vi "Choose configuration mode.vi"(8 "error in (no error)":errorcluster, 10 "Choose configuration mode":u16=65535, 11 "PS Control Actor in":refnum<class "PS Control Actor.lvclass">) -> (0 "error out":errorcluster, 3 "PS Control Actor out":refnum<class "PS Control Actor.lvclass">)   [LabVIEW 2025, in "PS Control Actor.lvlib" / "PS Control Actor.lvclass"]
doc: "Author: Scott Hannahs <sth@magnet.fsu.edu>\n\nThis software is licensed for use under the “MIT License\"\nCopyright (c) 2025 Scott Hannahs, sth@sth@magnet.sthnet.net\n\nPermission is hereby granted, free of charge, to any person obtaining a copy of this software and associated documentation files (the \"Software\"), to deal in the Software without restriction, including without limitation the rights to use, copy, modify, merge, publish, distribute, sublicense, and/or sell copies of the Software, and to permit persons to whom the Software is furnished to do so, subject to the following conditions: The above copyright notice and this permission notice shall be included in all copies or substantial portions of the Software.\n\nTHE SOFTWARE IS PROVIDED \"AS IS\", WITHOUT WARRANTY OF ANY KIND, EXPRESS OR IMPLIED, INCLUDING BUT NOT LIMITED TO THE WARRANTIES OF MERCHANTABILITY, FITNESS FOR A PARTICULAR PURPOSE AND NONINFRINGEMENT. IN NO EVENT SHALL THE AUTHORS OR COPYRIGHT HOLDERS BE LIABLE FOR ANY CLAIM, DAMAGES OR OTHER LIABILITY, WHETHER IN AN ACTION OF CONTRACT, TORT OR OTHERWISE, ARISING FROM, OUT OF OR IN CONNECTION WITH THE SOFTWARE OR THE USE OR OTHER DEALINGS IN THE SOFTWARE."
uses:
  PS Control Actor.lvclass
  PS Control Actor.lvclass/PS Control Actor.ctl
  PS Driver/PS Driver.lvclass
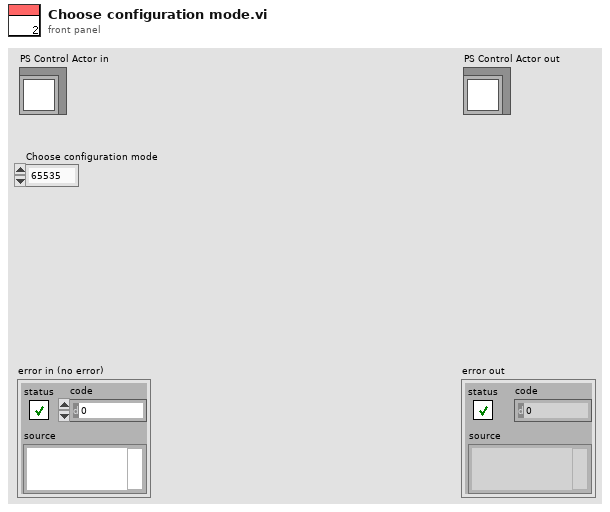
[diagram p1: front panel]
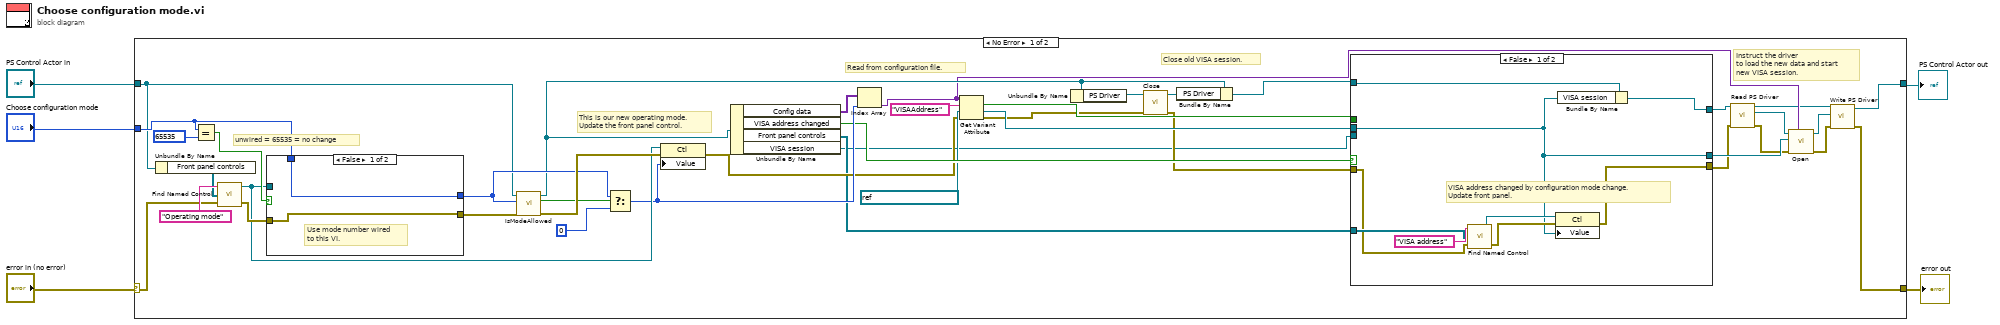
[diagram p0: block diagram]
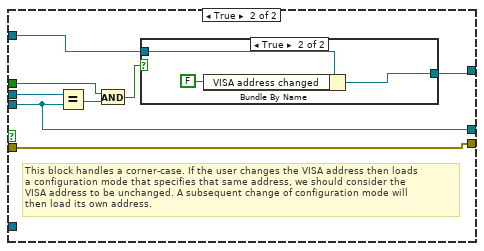
[diagram p2: hidden frame]
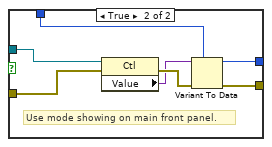
[diagram p4: hidden frame]
diagram:
  n1 = case shown="No Error" "error in (no error)" {
    selector: "error in (no error)" -> [w35 w78]
    tunnel: [w13 w78] -> w4
    tunnel: [w7 w77] -> w1
    tunnel: "PS Control Actor in" -> [w34 w77]
    tunnel: "Choose configuration mode" -> [w42 _]
    frame No Error {
      # "Close old VISA session."
      # "Read from configuration file."
      # "Instruct the driver \nto load the new data and start\nnew VISA session."
      # "This is our new operating mode.\nUpdate the front panel control."
      # "unwired = 65535 = no change"
      n2 = Unbundle By Name(w34) -> ("Front panel controls"=w33:refnum<vi>[])
      n3 = Equal?(x=w42, y=u16 65535) -> (x = y?=w45:bool)
      n4 = call "Find Named Control.vi"("error in"=w35, "All Controls"=w33, "Control Name"="Operating mode") -> ("error out"=w43:errorcluster, "Ctl Refnum"=w36:refnum<vi>)  [unwired: 1 out]
      n5 = case shown="False" w45 {
        tunnel: [w68 w74] -> w39
        tunnel: [w69 w73] -> w41
        tunnel: w43 -> [w69 w72]
        tunnel: w36 -> [_ w71]
        tunnel: w42 -> [w68 w70]
        frame False {
          # "Use mode number wired\nto this VI."
        }
        frame True {
          # "Use mode showing on main front panel."
          n6 = property class="Ctl"(reference=w71, error in=w72) -> (error out=w76:errorcluster, "Value"=w75:variant)  [unwired: 1 out]
          n7 = Variant To Data(error in=w76, type=w70, Variant=w75) -> (data=w74:u16, error out=w73:errorcluster)
        }
      }
      n8 = call "IsModeAllowed.vi"("error in (no error)"=w41, "Mode"=w39, "PS Control Actor in"=w34) -> ("error out"=w40:errorcluster, "Allowed"=w38:bool, "PS Control Actor out"=w23:refnum<class "PS Control Actor.lvclass">)  [unwired: 6 in]
      n9 = Select(t=w39, s=w38, f=u16 0) -> (s? t:f=w32:u16)
      n10 = property class="Ctl"(reference=w36, error in=w40, "Value"=w32) -> (error out=w20:errorcluster)  [unwired: 1 out]
      n11 = Unbundle By Name(w23) -> ("Config data"=w17:variant[], "VISA address changed"=w31:bool, "Front panel controls"=w19:refnum<vi>[], "VISA session"=w18:refnum<visa-resource-name>)
      n12 = Index Array(array=w17, index=w32) -> (element=w15:variant)
      n13 = Get Variant Attribute(Variant=w15, name="VISAAddress", default value (empty Variant)=refnum<visa-resource-name> "GPIB0::100::INSTR" ("VISA address 2"), error in=w20) -> (found=w29:bool, value=w28:refnum<visa-resource-name>, error out=w25:errorcluster)  [unwired: 1 out]
      n14 = Unbundle By Name(w23) -> ("PS Driver"=w26:refnum<class "PS Driver.lvclass">)
      n15 = call-dynamic "Close.vi"("error in (no error)"=w25, "PS Driver Actor in"=w26) -> ("error out"=w24:errorcluster, "PS Driver Actor out"=w21:refnum<class "PS Driver.lvclass">)  [unwired: 8 in]
      n16 = Bundle By Name(cluster=w23, "PS Driver"=w21) -> (w22:refnum<class "PS Control Actor.lvclass">)
      n17 = case shown="False" w31 {
        tunnel: w24 -> [w50 w57]
        tunnel: [w54 w57] -> w12
        tunnel: w22 -> [w53 w61]
        tunnel: [w55 w60] -> w9
        tunnel: w29 -> [_ w59]
        tunnel: w28 -> [w47 w58]
        tunnel: w18 -> [_ w56]
        tunnel: w19 -> [w51 _]
        tunnel: [w47 w56] -> w16
        frame False {
          # "VISA address changed by configuration mode change.\nUpdate front panel."
          n18 = call "Find Named Control.vi"("error in"=w50, "All Controls"=w51, "Control Name"="VISA address") -> ("error out"=w49:errorcluster, "Ctl Refnum"=w48:refnum<vi>)  [unwired: 1 out]
          n19 = property class="Ctl"(reference=w48, error in=w49, "Value"=w47) -> (error out=w54:errorcluster)  [unwired: 1 out]
          n20 = Bundle By Name(cluster=w53, "VISA session"=w47) -> (w55:refnum<class "PS Control Actor.lvclass">)
        }
        frame True {
          # "This block handles a corner-case. If the user changes the VISA address then loads\na configuration mode that specifies that same address, we should consider the\nVISA address to be unchanged. A subsequent change of configuration mode will\nthen load its own address."
          n21 = Equal?(x=w58, y=w56) -> (x = y?=w63:bool)
          n22 = And(x=w59, y=w63) -> (x .and. y?=w62:bool)
          n23 = case shown="True" w62 {
            tunnel: w61 -> [w64 w67]
            tunnel: [w64 w66] -> w60
            frame False {
            }
            frame True {
              n24 = Bundle By Name(cluster=w67, "VISA address changed"=FALSE) -> (w66:refnum<class "PS Control Actor.lvclass">)
            }
          }
        }
      }
      n25 = call-dynamic "Read PS Driver.vi"("error in (no error)"=w12, "PS Control Actor in"=w9) -> ("error out"=w11:errorcluster, "PS Driver.lvlib:PS Driver.lvclass"=w10:refnum<class "PS Driver.lvclass">, "PS Control Actor out"=w8:refnum<class "PS Control Actor.lvclass">)  [unwired: 7 in]
      n26 = call-dynamic "Open.vi"("Config data in"=w15, "error in (no error)"=w11, "VISA session"=w16, "PS Driver.lvlib:PS Driver.lvclass in"=w10) -> ("error out"=w14:errorcluster, "PS Driver.lvlib:PS Driver.lvclass out"=w6:refnum<class "PS Driver.lvclass">)  [unwired: 4 in, 2 out]
      n27 = call-dynamic "Write PS Driver.vi"("error in (no error)"=w14, "PS Driver.lvlib:PS Driver.lvclass"=w6, "PS Control Actor in"=w8) -> ("error out"=w13:errorcluster, "PS Control Actor out"=w7:refnum<class "PS Control Actor.lvclass">)  [unwired: 7 in]
    }
    frame Error {
    }
  }
  "error out" <- w4
  "PS Control Actor out" <- w1
